vi "PutFile.vi"(8 "error in (no error)":errorcluster) -> (0 "error out":errorcluster, 2 "Serverpath":string)   [LabVIEW 2024, in "FTPS.lvlib"]
doc: "This VI : Put File\n------------------------------------------------------------------------------------------\nTransfers the file from \"FTP Client \" to \"FTP Server\"\n------------------------------------------------------------------------------------------\n-FilePath(Remote) - Pass the file path ie on FTP server , where file need to be transfer.\n-FilePath(NeedToBeSent) -Pass the file path of the file i.e. need to be transfer."
uses:
  FTPS.lvlib
  <vilib>/Utility/file.llb/Read Delimited Spreadsheet (string).vi
  <vilib>/Utility/file.llb/Write Delimited Spreadsheet (string).vi
  <vilib>/FTP/NI_FTP.lvlib
  Launcher/Launcher_DTU.lvlib
panel:
  in  "FilePath(Remote)":string="/River/"
  in  "FilePath(NeedTobeSent)":path=path "C:/FTPLocal/ssl_config_1.csv"
  in  "ClusterSetting":T1={"password"="1234", "user"="ftpadmin", "remote path"="/River/ssl_config.csv", "host"="169.254.73.100"}
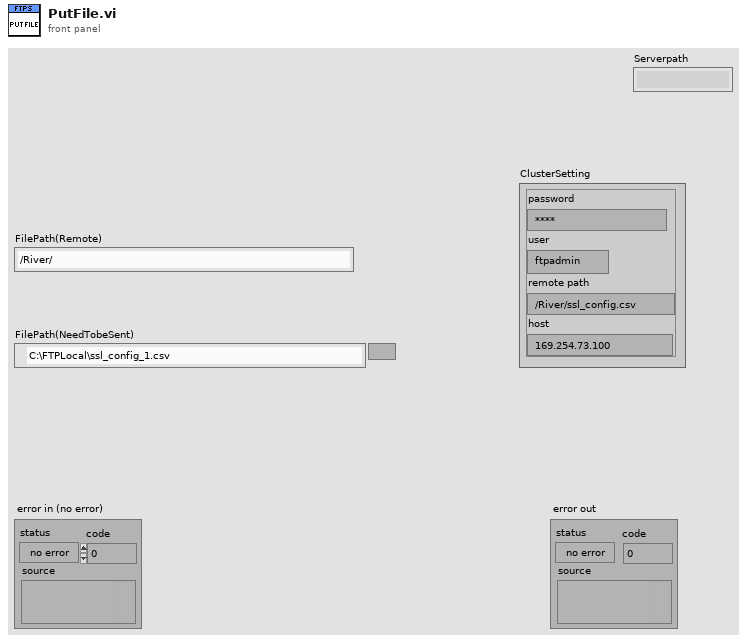
[diagram p1: front panel]
types:
  T1 = cluster{"password":string, "user":string, "remote path":string, "host":string}
  T2 = enum16{"open", "replace", "create", "open or create", "replace or create", "replace or create with confirmation"}
  T3 = enum16{"Read", "Write", "All_sections", "All_values", "Remove key&section"}
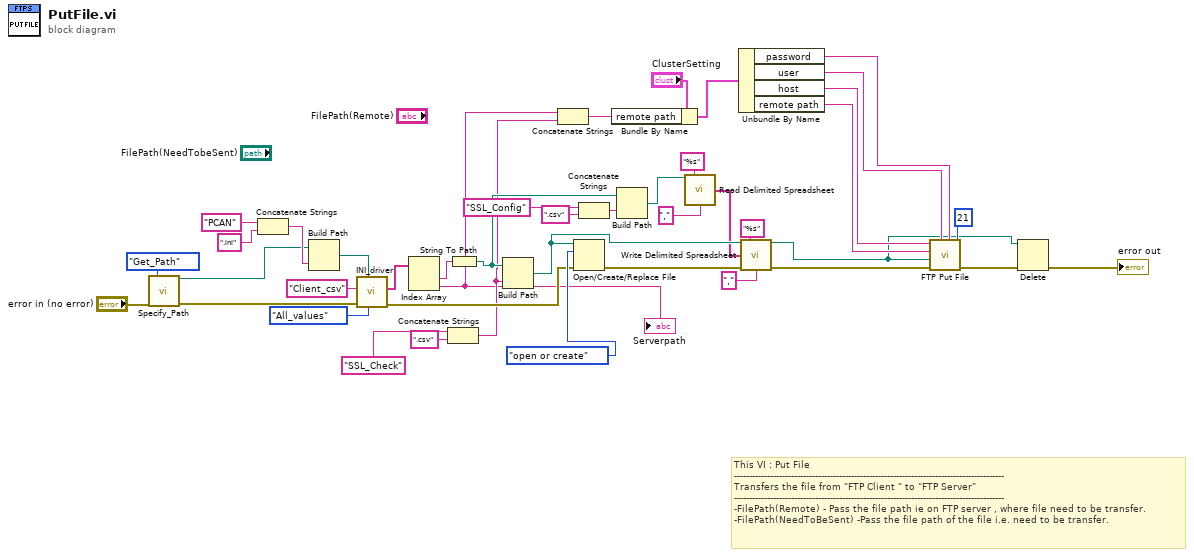
[diagram p0: block diagram]
diagram:
  # "This VI : Put File\n------------------------------------------------------------------------------------------\nTransfers the file from \"FTP Client \" to \"FTP Server\"\n------------------------------------------------------------------------------------------\n-FilePath(Remote) - Pass the file path ie on FTP server , where file need to be transfer.\n-FilePath(NeedToBeSent) -Pass the file path of the file i.e. need to be transfer."
  n1 = call "Specify_Path.vi"("Path_Enum"=enum16{"Find_Path", "Get_Path"}."Get_Path", "error in (no error)"="error in (no error)") -> ("Configurations"=w26:path, "error out"=w30:errorcluster)  [unwired: 6 in, 6 out]
  n2 = Concatenate Strings("PCAN" ("string"), ".ini" ("string")) -> (w32:string)
  n3 = Build Path(base path=w26, name or relative path=w32) -> (appended path=w31:path)
  n4 = call "INI_driver.vi"("Enum"=T3."All_values", "instrument file path"=w31, "error in (no error)"=w30, "Section"="Client_csv") -> ("error out"=w21:errorcluster, "Values out"=w24:string[])  [unwired: 4 in, 2 out]
  n5 = Index Array(array=w24) -> (element #1=w23:string, element #2=w2:string)  [unwired: 2 in]
  "Serverpath" <- w2
  n6 = Concatenate Strings("SSL_Check", ".csv" ("string")) -> (w13:string)
  n7 = String To Path(string=w23) -> (path=w18:path)
  n8 = Build Path(base path=w18, name or relative path=w13) -> (appended path=w11:path)
  n9 = Concatenate Strings(w2, w13) -> (w14:string)
  n10 = Open/Create/Replace File(file path (use dialog)=w11, error in=w21, operation (0:open)=T2."open or create") -> (error out=w19:errorcluster)  [unwired: 3 in, 2 out]
  n11 = Concatenate Strings("SSL_Config" ("string"), ".csv" ("string")) -> (w16:string)
  n12 = Bundle By Name(cluster="ClusterSetting", "remote path"=w14) -> (w35:T1)
  n13 = Build Path(base path=w18, name or relative path=w16) -> (appended path=w10:path)
  n14 = call-poly <vilib>:"Read Delimited Spreadsheet.vi"("file path (dialog if empty)"=w10, "format (%s)"="%s", "delimiter (\\t)"="," ("delimiter (\\t)")) -> ("first row"=w7:string[])  [unwired: 7 in, 5 out]
  n15 = Unbundle By Name(w35) -> ("password"=w41:string, "user"=w40:string, "host"=w39:string, "remote path"=w38:string)
  n16 = call-poly <vilib>:"Write Delimited Spreadsheet.vi"("file path (dialog if empty)"=w11, "format (%s)"="%s" ("format (%.3f)"), "1D data"=w7, "error in (no error)"=w19, "delimiter (\\t)"="," ("delimiter (\\t)")) -> ("new file path (Not A Path if cancelled)"=w3:path, "error out"=w12:errorcluster)  [unwired: 9 in]
  n17 = call <vilib>:"FTP Put File.vi"("remote port (21)"=u16 21, "password"=w41, "user"=w40, "error in (no error)"=w12, "local path"=w3, "remote path"=w38, "host"=w39) -> ("error out"=w37:errorcluster)  [unwired: 3 in, 1 out]
  n18 = Delete(path (use dialog)=w3, error in=w37) -> (error out=→"error out":errorcluster)  [unwired: 3 in, 2 out]
